vi "GFITS_ReadValueFromCtrl.vi"(0 "Vi name":string, 5 "Control Name":string, 7 "Type":string, 11 "error in":errorcluster) -> (4 "Value":string, 6 "value type":u16, 15 "error out":errorcluster)   [LabVIEW 2016]
panel:
  in  "Types":string[](array[string])=["STR", "BOOL", "EXT", "DBL", "SGL", "I32", "I16", "I8", "U32", "U16", "U8", "FGEnum", "Path"]
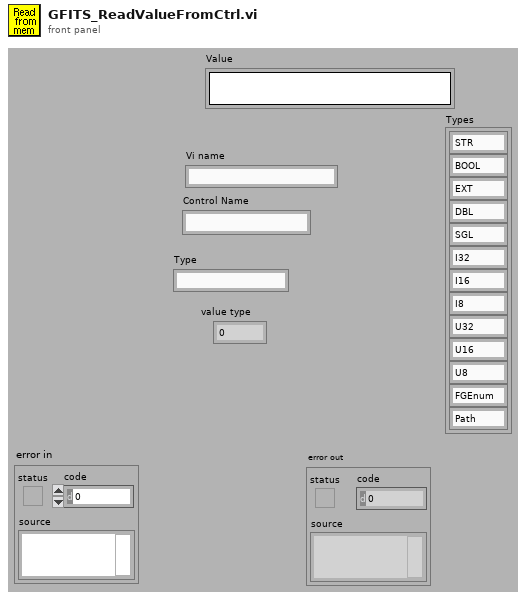
[diagram p1: front panel]
types:
  T1 = enum32{"Setup", "Settings", "Memory", "Utility", "Imaging", "Errors & Messages"}
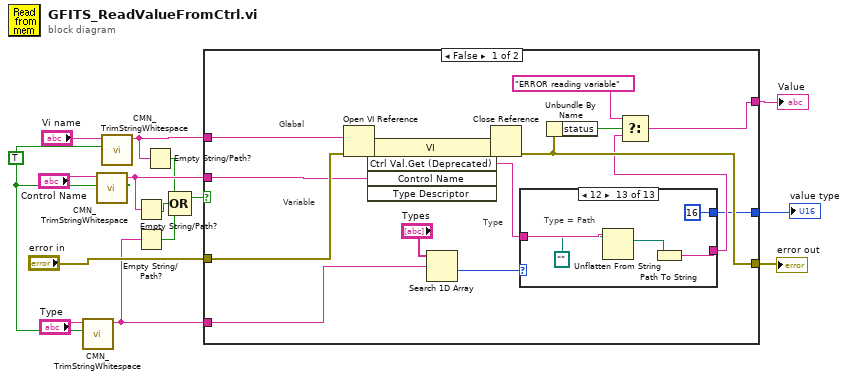
[diagram p0: block diagram]
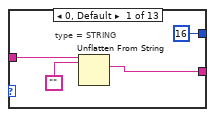
[diagram p2: hidden frame]
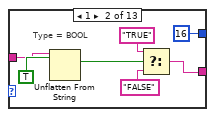
[diagram p3: hidden frame]
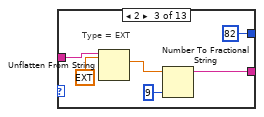
[diagram p4: hidden frame]
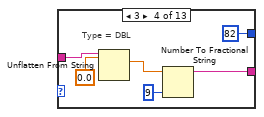
[diagram p5: hidden frame]
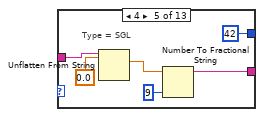
[diagram p6: hidden frame]
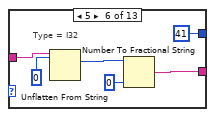
[diagram p7: hidden frame]
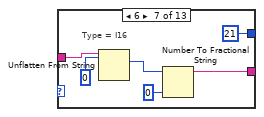
[diagram p8: hidden frame]
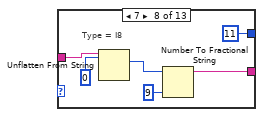
[diagram p9: hidden frame]
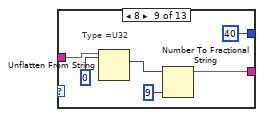
[diagram p10: hidden frame]
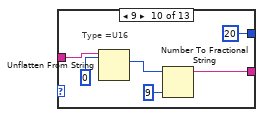
[diagram p11: hidden frame]
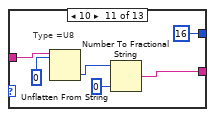
[diagram p12: hidden frame]
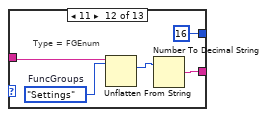
[diagram p13: hidden frame]
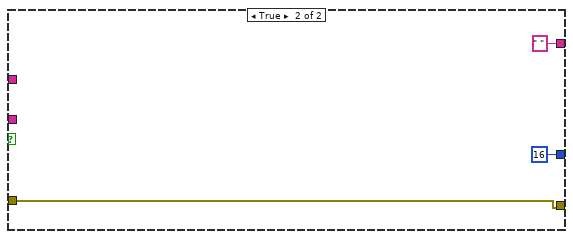
[diagram p14: hidden frame]
diagram:
  w9 = TRUE
  n1 = call "CMN_TrimStringWhitespace.vi"("Both Ends?(T)"=w9, "string"="Type") -> ("trimmed string"=w6:string)  [unwired: 8 out]
  n2 = call "CMN_TrimStringWhitespace.vi"("Both Ends?(T)"=w9, "string"="Control Name") -> ("trimmed string"=w7:string)  [unwired: 8 out]
  n3 = call "CMN_TrimStringWhitespace.vi"("Both Ends?(T)"=w9, "string"="Vi name") -> ("trimmed string"=w8:string)  [unwired: 8 out]
  n4 = Empty String/Path?(string/path=w7) -> (empty?=w4:bool)
  n5 = Empty String/Path?(string/path=w6) -> (empty?=w5:bool)
  n6 = Empty String/Path?(string/path=w8) -> (empty?=w3:bool)
  n7 = Compound Arithmetic op=OR(w3, w4, w5) -> (w2:bool)
  n8 = case shown="False" w2 {
    tunnel: [w32 w110] -> w15
    tunnel: [w31 " "] -> w14
    tunnel: "error in" -> [w30 w110]
    tunnel: w8 -> [w19 _]
    tunnel: w7 -> [w18 _]
    tunnel: w6 -> [w17 _]
    tunnel: [w16 16] -> w1
    frame False {
      # "Type"
      # "Variable"
      # "Glabal"
      n9 = Open VI Reference(vi path=w19, error in (no error)=w30) -> (vi reference=w28:refnum<vi>, error out=w29:errorcluster)  [unwired: 4 out]
      n10 = invoke class="VI" method="Ctrl Val.Get (Deprecated)"(reference=w28, error in=w29, "Control Name"=w18) -> (reference out=w26:refnum<vi>, error out=w27:errorcluster, "Get Control Value"=w25:string)  [unwired: 2 in, 2 out]
      n11 = Search 1D Array(1D array="Types", element=w17) -> (index of element=w24:i32)  [unwired: 1 out]
      n12 = Close Reference(reference=w26, error in (no error)=w27) -> (error out=w32:errorcluster)
      n13 = case shown="12" w24 {
        tunnel: w25 -> [w35 w42 w48 w54 w60 w66 w72 w78 w84 w90 w96 w102 w107]
        tunnel: [w34 w38 w45 w51 w57 w64 w69 w75 w81 w87 w94 w100 w104] -> w22
        tunnel: [16 16 82 82 42 41 21 11 40 20 16 16 16] -> w16
        frame 0, Default {
          # "type = STRING"
          n14 = Unflatten From String(type="", binary string=w35) -> (value=w34:string)  [unwired: 1 in, 4 out]
        }
        frame 1 {
          # "Type = BOOL"
          n15 = Unflatten From String(type=TRUE, binary string=w42) -> (value=w41:bool)  [unwired: 1 in, 4 out]
          n16 = Select(t="TRUE", s=w41, f="FALSE") -> (s? t:f=w38:string)
        }
        frame 2 {
          # "Type = EXT"
          n17 = Unflatten From String(type=ext 0.0, binary string=w48) -> (value=w47:ext)  [unwired: 1 in, 4 out]
          n18 = Number To Fractional String(number=w47, precision (6)=i16 9) -> (F-format string=w45:string)  [unwired: 2 out]
        }
        frame 3 {
          # "Type = DBL"
          n19 = Unflatten From String(type=0.0, binary string=w54) -> (value=w53:dbl)  [unwired: 1 in, 4 out]
          n20 = Number To Fractional String(number=w53, precision (6)=i16 9) -> (F-format string=w51:string)  [unwired: 2 out]
        }
        frame 4 {
          # "Type = SGL"
          n21 = Unflatten From String(type=sgl 0.0, binary string=w60) -> (value=w59:sgl)  [unwired: 1 in, 4 out]
          n22 = Number To Fractional String(number=w59, precision (6)=i16 9) -> (F-format string=w57:string)  [unwired: 2 out]
        }
        frame 5 {
          # "Type = I32"
          n23 = Unflatten From String(type=0, binary string=w66) -> (value=w65:i32)  [unwired: 1 in, 4 out]
          n24 = Number To Fractional String(number=w65, precision (6)=i16 0) -> (F-format string=w64:string)  [unwired: 2 out]
        }
        frame 6 {
          # "Type = I16"
          n25 = Unflatten From String(type=i16 0, binary string=w72) -> (value=w71:i16)  [unwired: 1 in, 4 out]
          n26 = Number To Fractional String(number=w71, precision (6)=i16 0) -> (F-format string=w69:string)  [unwired: 2 out]
        }
        frame 7 {
          # "Type = I8"
          n27 = Unflatten From String(type=i8 0, binary string=w78) -> (value=w77:i8)  [unwired: 1 in, 4 out]
          n28 = Number To Fractional String(number=w77, precision (6)=i16 9) -> (F-format string=w75:string)  [unwired: 2 out]
        }
        frame 8 {
          # "Type =U32"
          n29 = Unflatten From String(type=u32 0, binary string=w84) -> (value=w83:u32)  [unwired: 1 in, 4 out]
          n30 = Number To Fractional String(number=w83, precision (6)=i16 9) -> (F-format string=w81:string)  [unwired: 2 out]
        }
        frame 9 {
          # "Type =U16"
          n31 = Unflatten From String(type=u16 0, binary string=w90) -> (value=w89:u16)  [unwired: 1 in, 4 out]
          n32 = Number To Fractional String(number=w89, precision (6)=i16 9) -> (F-format string=w87:string)  [unwired: 2 out]
        }
        frame 10 {
          # "Type =U8"
          n33 = Unflatten From String(type=u8 0, binary string=w96) -> (value=w95:u8)  [unwired: 1 in, 4 out]
          n34 = Number To Fractional String(number=w95, precision (6)=i16 0) -> (F-format string=w94:string)  [unwired: 2 out]
        }
        frame 11 {
          w101 = T1."Settings"  # FuncGroups
          # "Type = FGEnum"
          n35 = Unflatten From String(type=w101, binary string=w102) -> (value=w99:T1)  [unwired: 1 in, 4 out]
          n36 = Number To Decimal String(number=w99) -> (decimal integer string=w100:string)  [unwired: 1 out]
        }
        frame 12 {
          # "Type = Path"
          n37 = Unflatten From String(type=path "", binary string=w107) -> (value=w105:path)  [unwired: 1 in, 4 out]
          n38 = Path To String(path=w105) -> (string=w104:string)
        }
      }
      n39 = Unbundle By Name(w32) -> ("status"=w23:bool)
      n40 = Select(t="ERROR reading variable", s=w23, f=w22) -> (s? t:f=w31:string)
    }
    frame True {
    }
  }
  "error out" <- w15
  "Value" <- w14
  "value type" <- w1
